vi "IsLVClass.vi"(3 "ProjectItem Refnum":refnum<vi>) -> (1 "IsLVClass?":bool)   [LabVIEW 2014, in "_ProjectItemsUtilities.lvlib"]
uses:
  _ProjectItemsUtilities.lvlib
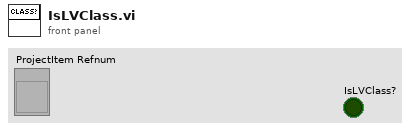
[diagram p1: front panel]
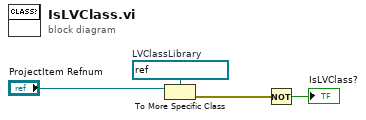
[diagram p0: block diagram]
diagram:
  w4 = refnum<vi> refnum  # LVClassLibrary
  n1 = To More Specific Class(target class=w4, reference="ProjectItem Refnum") -> (error out=w3:errorcluster)  [unwired: 1 in, 1 out]
  n2 = Not(x=w3) -> (.not. x?=→"IsLVClass?":bool)
